vi "RSZVB Set External Signal Source.vi"(8 "error in (no error)":errorcluster {"code" format="%.0x"}, 9 "External Signal Source (0)":i32, 10 "Channel (1)":i32=1, 11 "VISA session":refnum<visa-resource-name>) -> (0 "error out":errorcluster {"code" format="%.0x"}, 3 "dup VISA session":refnum<visa-resource-name>)   [LabVIEW 2011]
doc: "This VI sets an external generator as a signal source for the LO signal (external source).\n\nNotes:\n\n(0) Generators must be configured explicitly in the System - System Config - Configure External Generators VI.\n\nRemote-control command(s):\n[SENSe<Ch>:]FREQuency:CONVersion:MIXer:LOEXternal NONE | <port_number>"
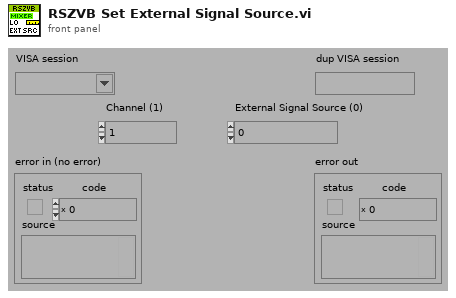
[diagram p1: front panel]
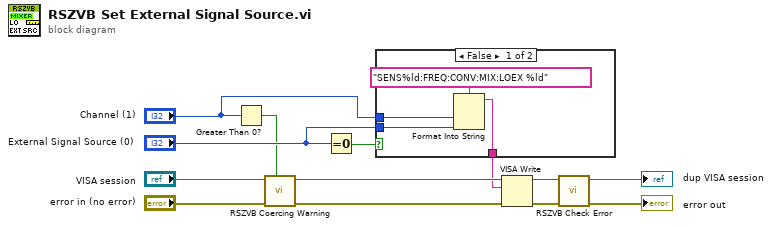
[diagram p0: block diagram]
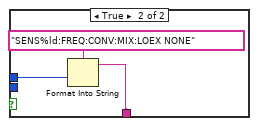
[diagram p2: hidden frame]
diagram:
  n1 = Greater Than 0?(x="Channel (1)") -> (x > 0?=w1:bool)
  n2 = call "RSZVB Coercing Warning.vi"("In Range?"=w1, "error in (no error)"="error in (no error)", "VISA session"="VISA session") -> ("error out"=w12:errorcluster, "dup VISA session"=w13:refnum<visa-resource-name>)  [unwired: 7 in]
  n3 = Equal To 0?(x="External Signal Source (0)") -> (x = 0?=w7:bool)
  n4 = case shown="False" w7 {
    tunnel: [w16 w18] -> w9
    tunnel: "Channel (1)" -> [w15 w19]
    tunnel: "External Signal Source (0)" -> [w14 _]
    frame False {
      n5 = Format Into String(format string="SENS%ld:FREQ:CONV:MIX:LOEX %ld", w15, w14) -> (resulting string=w16:string)  [unwired: 2 in, 1 out]
    }
    frame True {
      n6 = Format Into String(format string="SENS%ld:FREQ:CONV:MIX:LOEX NONE", w19) -> (resulting string=w18:string)  [unwired: 2 in, 1 out]
    }
  }
  n7 = VISA Write(VISA resource name=w13, write buffer=w9, error in (no error)=w12) -> (VISA resource name out=w10:refnum<visa-resource-name>, error out=w11:errorcluster)  [unwired: 1 out]
  n8 = call "RSZVB Check Error.vi"("error in (no error)"=w11, "VISA session"=w10) -> ("error out"=→"error out":errorcluster, "dup VISA session"=→"dup VISA session":refnum<visa-resource-name>)  [unwired: 8 in]
